vi "HB_Simple.Main.vi"() -> ()   [LabVIEW 2009, in "HB_BaseClass_Examples.lvlib"]
doc: "Simple demo VI."
uses:
  HB_BaseClass_Examples.lvlib
  HB_Simple.lvclass
  HB_Factory/HB_Factory.lvclass
  lib.lib/HGF_LVC/HGF_BaseClasses/HGF_Factory/HGF_Factory.lvclass
  lib.lib/HGF_LVC/HGF_Auxiliary/HGF_Auxiliary.lvlib
panel:
  in  "objectName":string
  out "initData found?":bool
  in  "Use Factory?":bool
  out "className":string
  out "objectName":string
  out "initialized?":bool
  out "createdFromFactory?":bool
  out "success":bool
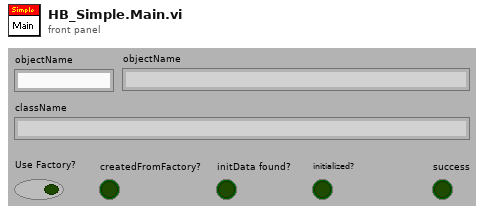
[diagram p1: front panel]
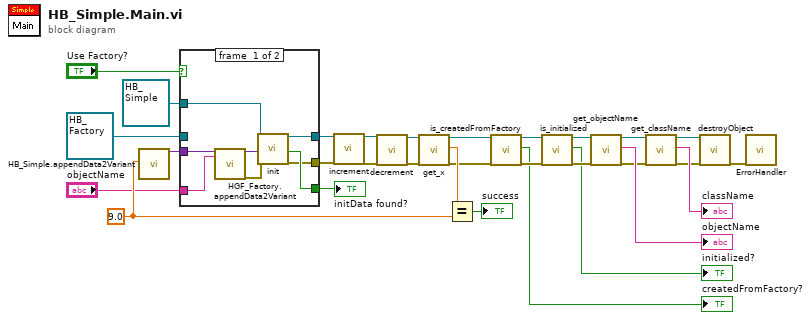
[diagram p0: block diagram]
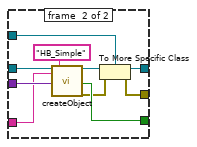
[diagram p2: hidden frame]
diagram:
  w21 = 9.0 ("x")
  n1 = call "HB_Simple.appendData2Variant.vi"("x"=w21) -> ("dup initData"=w30:variant)  [unwired: 17 in, 1 out]
  n2 = case shown="True" "Use Factory?" {
    tunnel: w30 -> [w38 w47]
    tunnel: [w37 w45] -> w29
    tunnel: [w35 w42] -> w28
    tunnel: refnum<class "HB_Simple.lvclass"> refnum ("HGF_BaseClass_Examples.lvlib:HB_Simple.lvclass") -> [w32 w43]
    tunnel: [w36 w46] -> w6
    tunnel: refnum<class "HB_Factory.lvclass"> refnum ("HB_HGF_Test.lvlib:HB_Factory.lvclass") -> [_ w41]
    tunnel: "objectName" -> [w31 w40]
    frame #0 {
      n3 = call "HGF_Factory.appendData2Variant.vi"("initData"=w38, "objectName"=w31) -> ("dup initData"=w33:variant, "error out"=w34:errorcluster)  [unwired: 3 in, 13 out]
      n4 = call "init.vi"("HGF_Object"=w32, "initializationData"=w33, "error in (no error)"=w34) -> ("dup HGF_Object"=w37:refnum<class "HB_Simple.lvclass">, "found?"=w36:bool, "error out"=w35:errorcluster)  [unwired: 14 out]
    }
    frame #1 {
      n5 = call "createObject.vi"("HGF_Factory"=w41, "objectName"=w40, "initializationData"=w47, "className"="HB_Simple") -> ("HGF_Object"=w39:refnum<class "HGF_Factory.lvclass">, "found?"=w46:bool, "error out"=w44:errorcluster)  [unwired: 1 in, 12 out]
      n6 = To More Specific Class(target class=w43, reference=w39, error in=w44) -> (specific class reference=w45:refnum<class "HB_Simple.lvclass">, error out=w42:errorcluster)
    }
  }
  "initData found?" <- w6
  n7 = call "increment.vi"("HB_Simple in"=w29, "error in (no error)"=w28) -> ("HB_Simple out"=w26:refnum<class "HB_Simple.lvclass">, "error out"=w25:errorcluster)  [unwired: 16 out]
  n8 = call "decrement.vi"("HB_Simple in"=w26, "error in (no error)"=w25) -> ("HB_Simple out"=w23:refnum<class "HB_Simple.lvclass">, "error out"=w24:errorcluster)  [unwired: 16 out]
  n9 = call "get_x.vi"("HB_Simple"=w23, "error in (no error)"=w24) -> ("dup HB_Simple"=w19:refnum<class "HB_Simple.lvclass">, "x"=w22:dbl, "error out"=w18:errorcluster)  [unwired: 15 out]
  n10 = Equal?(x=w22, y=w21) -> (x = y?=→"success":bool)
  n11 = call "is_createdFromFactory.vi"("HGF_Factory"=w19, "error in (no error)"=w18) -> ("dup HGF_Factory"=w17:refnum<class "HB_Simple.lvclass">, "createdFromFactory?"=→"createdFromFactory?":bool, "error out"=w16:errorcluster)  [unwired: 15 out]
  n12 = call "is_initialized.vi"("HGF_Factory"=w17, "error in (no error)"=w16) -> ("dup HGF_Factory"=w15:refnum<class "HB_Simple.lvclass">, "initialized?"=→"initialized?":bool, "error out"=w14:errorcluster)  [unwired: 15 out]
  n13 = call "get_objectName.vi"("HGF_Factory"=w15, "error in (no error)"=w14) -> ("dup HGF_Factory"=w10:refnum<class "HB_Simple.lvclass">, "objectName"=→"objectName":string, "error out"=w9:errorcluster)  [unwired: 15 out]
  n14 = call "get_className.vi"("HGF_Factory"=w10, "error in (no error)"=w9) -> ("dup HGF_Factory"=w3:refnum<class "HB_Simple.lvclass">, "className"=→"className":string, "error out"=w2:errorcluster)  [unwired: 15 out]
  n15 = call "destroyObject.vi"("HGF_Factory"=w3, "error in (no error)"=w2) -> ("error out"=w1:errorcluster)  [unwired: 17 out]
  n16 = call "ErrorHandler.vi"("error in (no error)"=w1) -> ()  [unwired: 6 in, 13 out]
